vi "Track3.vi"() -> ()   [LabVIEW 2011]
doc: "This VI demonstrates how to control the Robotics Starter Kit 1.0 robot. It is deployed to an sbRIO-9631, then run on the Real-Time controller."
uses:
  <vilib>/Analysis/Matrix/Datatypes/RealMatrix.ctl
  <vilib>/Platform/TimedLoop/XDataNode/timing_clust.ctl
  <vilib>/Platform/TimedLoop/XDataNode/nitl_modes.ctl
  <vilib>/Platform/TimedLoop/XDataNode/wakeup.ctl
  <vilib>/robotics/Starter Kit/1.0/9631 Host Interface/NI_Robotics_Starter Kit Host_9631_1.0.lvclass
  <vilib>/Analysis/Matrix/Numeric/Conversions/Array To Matrix - RA.vi
  <vilib>/Platform/TimedLoop/XDataNode/XDataNode.xnode
  <vilib>/Platform/TimedLoop/XDataNode/XDNodeRunTimeDep.lvlib
  <vilib>/Analysis/Matrix/NI_Matrix.lvlib
  <vilib>/robotics/Starter Kit/Host Interface/NI_Robotics_Starter Kit Host.lvclass
panel:
  out "X-Y 4":cluster{dbl[], dbl[]}(graph)
  out "W":cluster{dbl[], dbl[]}(graph)
  out "VL":cluster{dbl[], dbl[]}(graph)
  in  "Kp W":dbl step=0.01
  in  "Kp VL":dbl step=0.01
  in  "Paso":dbl
  in  "Tiempo":dbl
  in  "stop":bool
  out "X-Y":cluster{dbl[], dbl[]}(graph)
  out "Error":T1
  out "Xr - X":dbl[](array[numeric])
  out "Zigma":dbl[](array[numeric])
  out "Zigmar":dbl[](array[numeric])
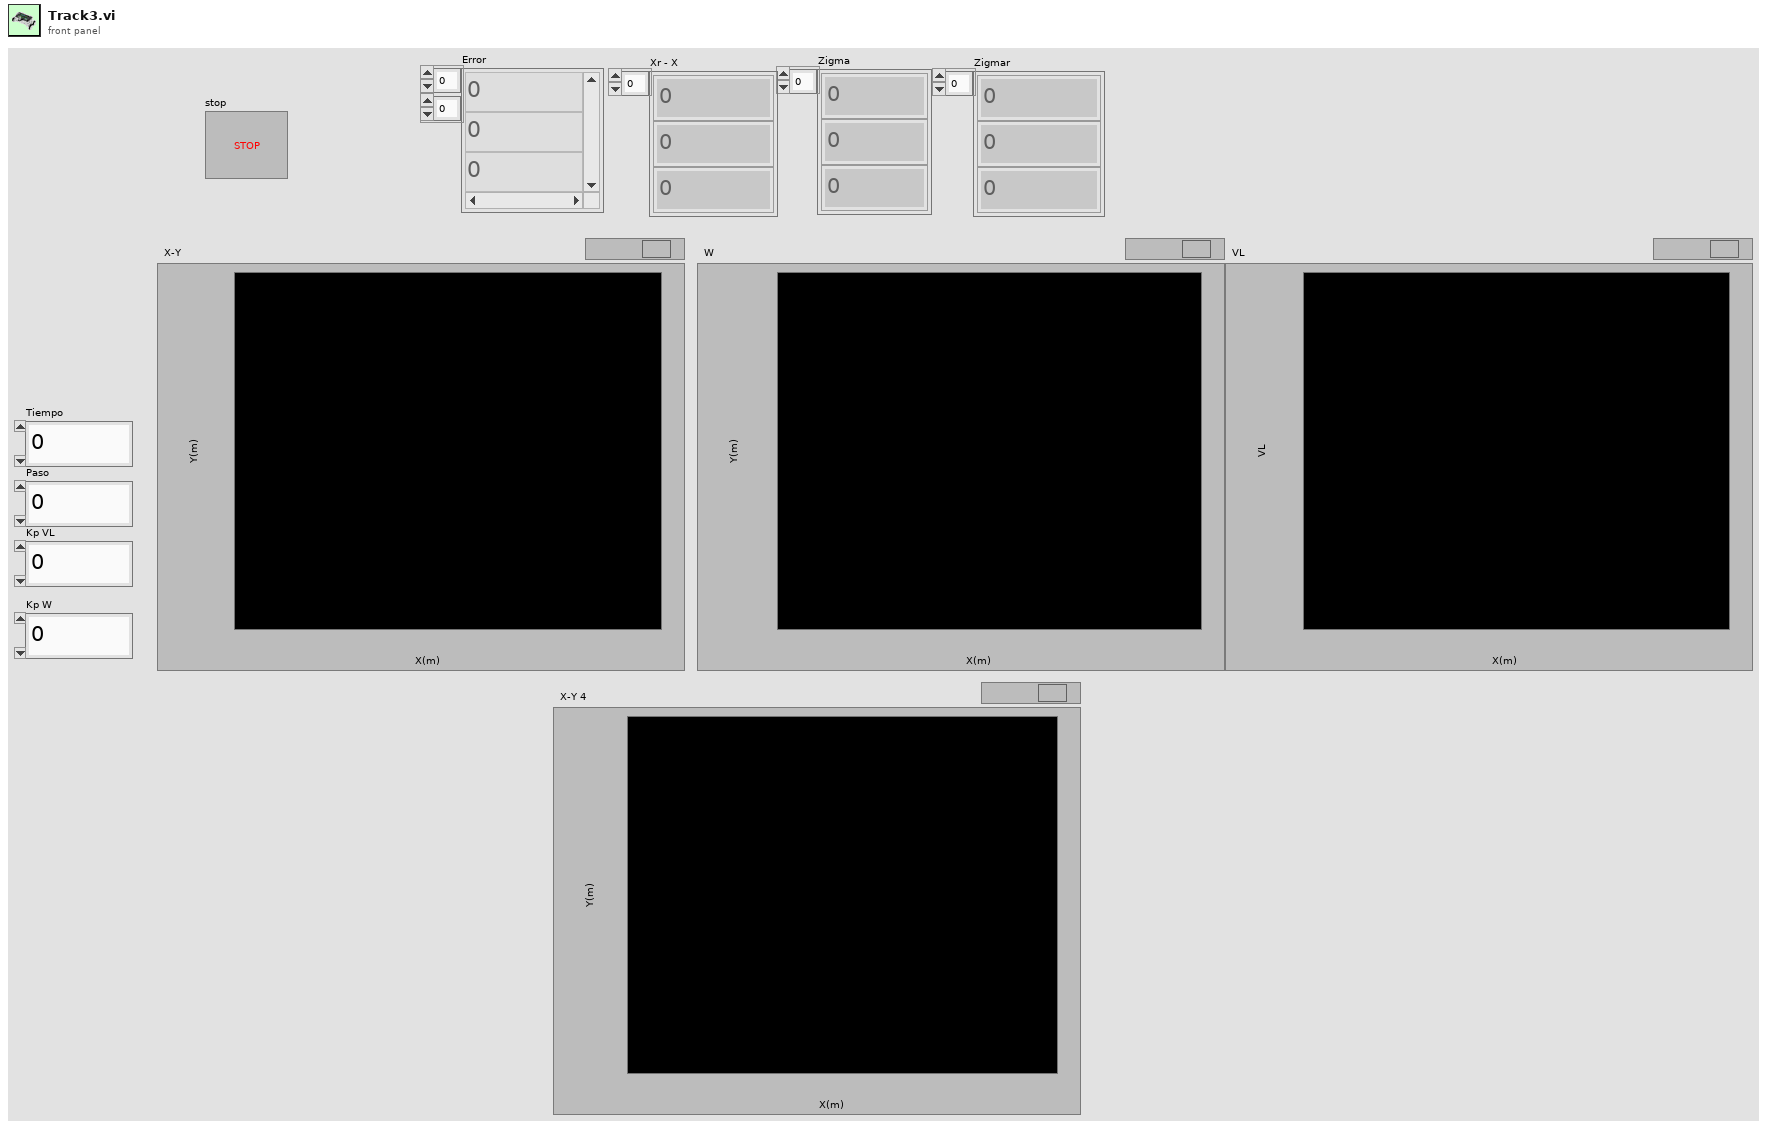
[diagram p1: front panel]
types:
  T1 = typedef "NI_Matrix.lvlib/RealMatrix.ctl" = dbl[][]
  T2 = typedef "XDNodeRunTimeDep.lvlib/timing_clust.ctl" = cluster{"Expected End [f-1]":u64, "Actual End [f-1]":u64, "Finished Late? [f-1]":bool, "Expected End [i-1]":u64, "Actual End [i-1]":u64, "Finished Late? [i-1]":bool, "Expected Start [i]":u64, "Actual Start [i]":u64, "Expected Start [f]":u64, "Actual Start [f]":u64, "Source Name":string, "Structure Name":string, "Period":i64, "Deadline":i64, "Offset":i64, "Start":i64, "Priority":i32, "Timeout":i32, "Mode":T3, "Wakeup Reason":T4, "Error":errorcluster, "Source Type":string, "Secondary Source Type":string, "Global End Time":u64, "Global Start Time":u64, "Frame Duration":u64, "Iteration Duration":u64, "Assigned CPU":i32, "I/O Scan Engine Mode":u32}
  T3 = typedef "XDNodeRunTimeDep.lvlib/nitl_modes.ctl" = enum32{"No Change", "Process missed periods, maintain original phase", "Discard missed periods, maintain original phase", "Process missed periods, ignore original phase", "Discard missed periods, ignore original phase"}
  T4 = typedef "XDNodeRunTimeDep.lvlib/wakeup.ctl" = enum32{"Normal", "Aborted", "Asynchronous wakeup", "Timing source error", "Timed loop error", "Timeout"}
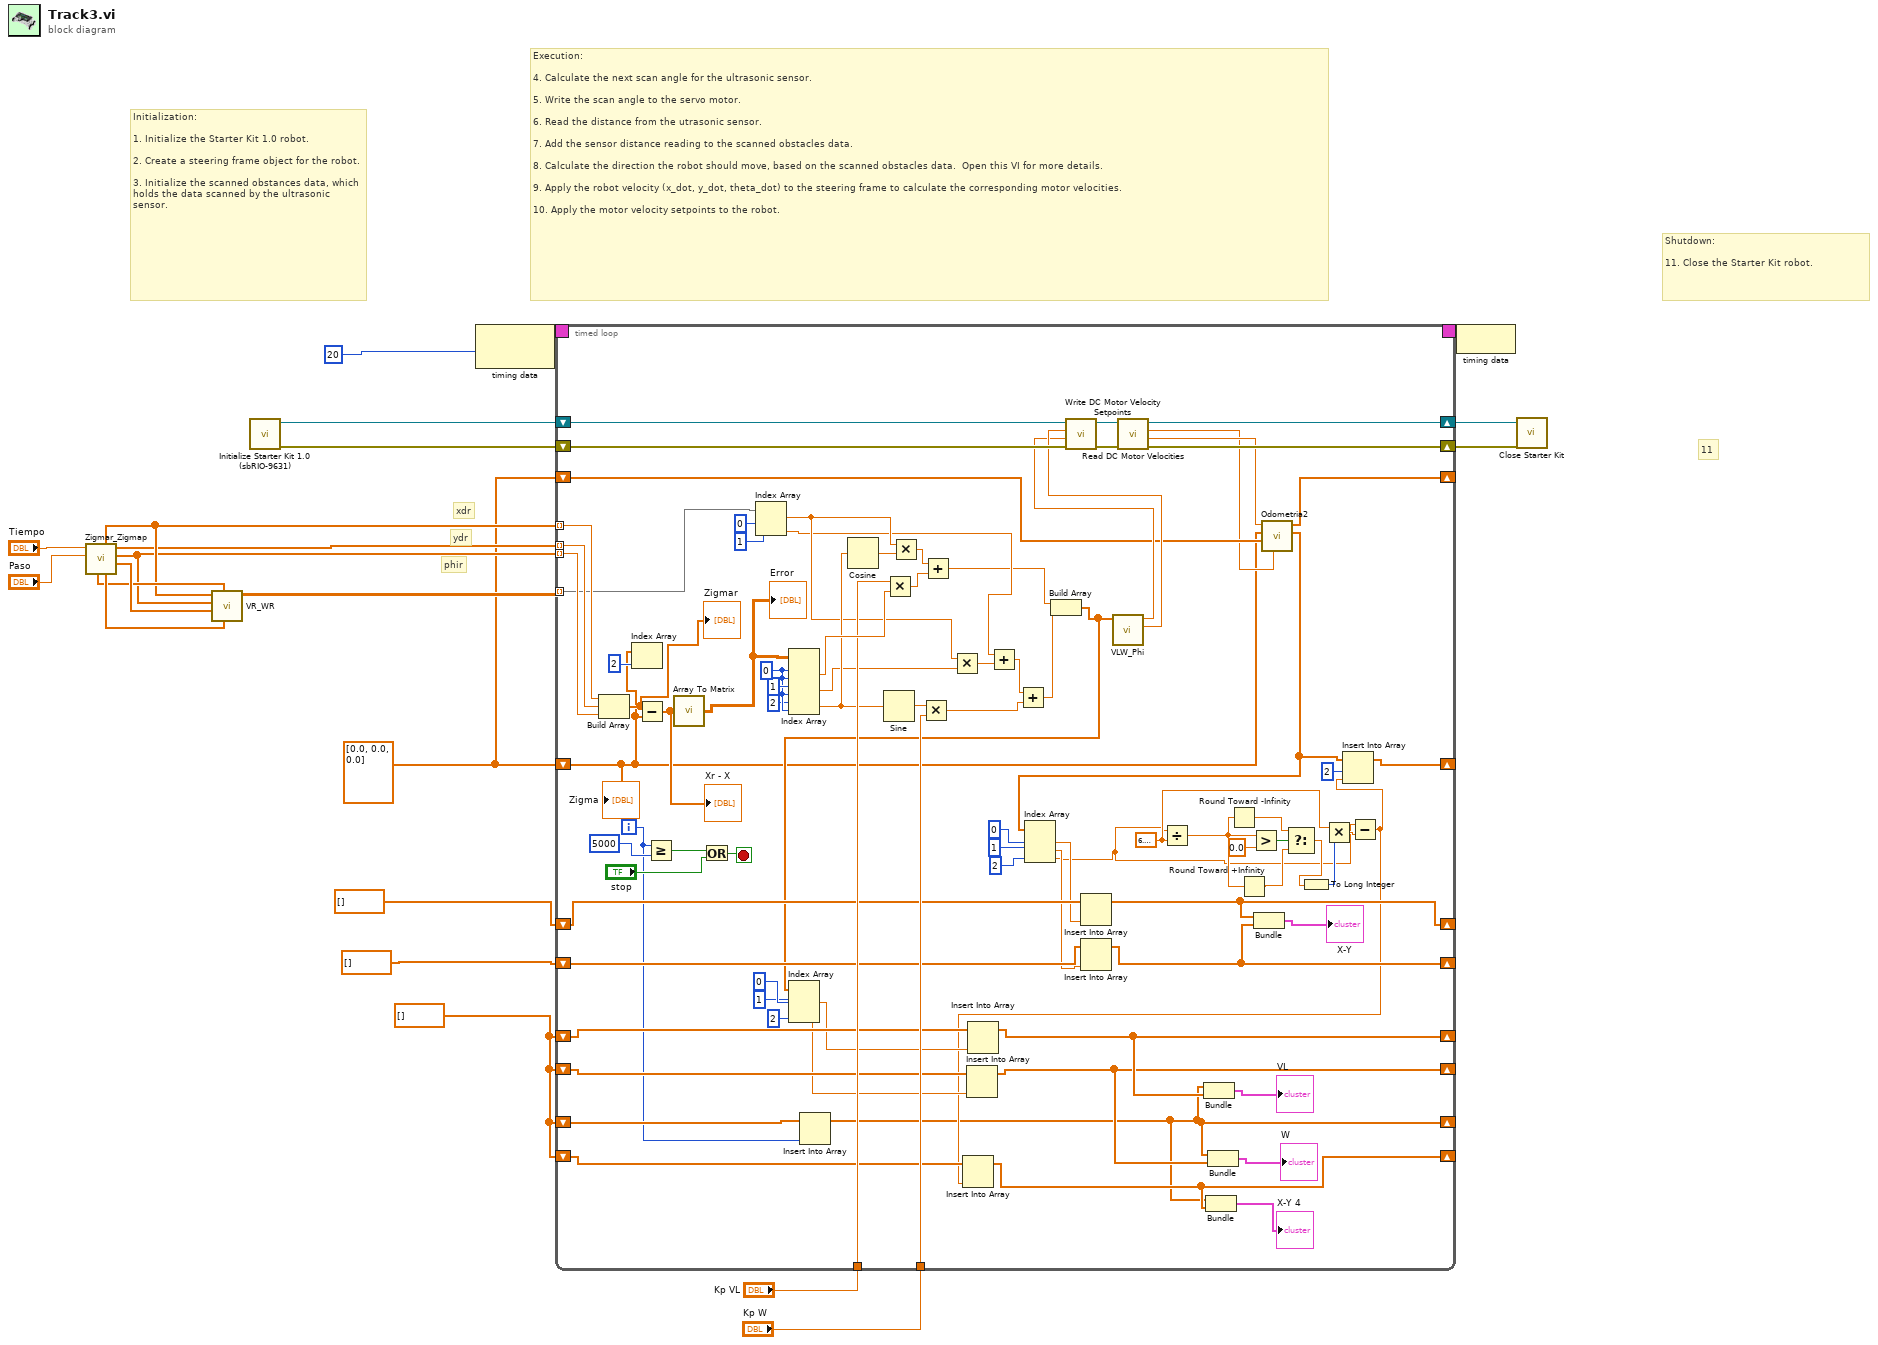
[diagram p0: block diagram]
diagram:
  w1 = dbl[] []
  w8 = dbl[] [0.0, 0.0, 0.0]
  # "phir"
  # "ydr"
  # "xdr"
  # "11"
  # "Shutdown:\n\n11. Close the Starter Kit robot."
  # "Execution:\n\n4. Calculate the next scan angle for the ultrasonic sensor.\n\n5. Write the scan angle to the servo motor.\n\n6. Read the distance from the utrasonic sensor.\n\n7. Add the sensor distance reading to the scanned obstacles data.\n\n8. Calculate the direction the robot should move, based on the scanned obstacles data.  Open this VI for more details.\n\n9. Apply the robot velocity (x_dot, y_dot, theta_dot) to the steering frame to calculate the corresponding motor velocities.\n\n10. Apply the motor velocity setpoints to the robot."
  # "Initialization:\n\n1. Initialize the Starter Kit 1.0 robot.\n\n2. Create a steering frame object for the robot.\n\n3. Initialize the scanned obstances data, which holds the data scanned by the ultrasonic sensor."
  n1 = call "Zigmar_Zigmap.vi"("Paso"="Paso", "Tiempo"="Tiempo") -> ("Xdrp"=w16:dbl[], "Phir"=w11:dbl[], "Ydr"=w12:dbl[], "Ydrp"=w17:dbl[], "Xdr"=w13:dbl[], "Phirp"=w15:dbl[])  [unwired: 4 in]
  n2 = call "VR_WR.vi"("Ydrp"=w17, "Phirp"=w15, "Xdrp"=w16, "Phir"=w11, "Xdr"=w13) -> ("Array"=w14:dbl[][])  [unwired: 6 in]
  n3 = call <vilib>:"Initialize Starter Kit 1.0 (sbRIO-9631).vi"() -> ("error out"=w5:errorcluster, "FPGA starter kit host 1.0 out"=w4:refnum<class "NI_Robotics_Starter Kit Host_9631_1.0.lvclass">)  [unwired: 10 in]
  n4 = node-c288(i64 20 ("Period")) -> (w22:T2)
  n5 = timed-loop {
    shift-right: [w77] -> w2
    shift-left: w4 -> [w79]
    shift-right: [w76] -> w3
    shift-left: w5 -> [w78]
    timing: w22 -> [_]
    timing-out: [_] -> w21
    tunnel: w14 -> [w101] mode=indexing
    tunnel: w13 -> [w110] mode=indexing
    tunnel: w12 -> [w109] mode=indexing
    tunnel: w11 -> [w108] mode=indexing
    shift-right: [w56] -> _
    shift-left: w8 -> [w24]
    tunnel: "Kp VL" -> [w96]
    tunnel: "Kp W" -> [w90]
    shift-right: [w70] -> _
    shift-left: w8 -> [w71]
    shift-right: [w63] -> _
    shift-left: dbl[] [] -> [w69]
    shift-right: [w62] -> _
    shift-left: dbl[] [] -> [w65]
    shift-right: [w35] -> _
    shift-left: w1 -> [w44]
    shift-right: [w30] -> _
    shift-left: w1 -> [w39]
    shift-right: [w26] -> _
    shift-left: w1 -> [w34]
    shift-right: [w29] -> _
    shift-left: w1 -> [w32]
    i -> [w33]
    stop <- w106 stop-if-true
    w55 = 6.283185307179586
    w99 = 0 ("index (row)")
    n6 = Build Array(w110, w109, w108) -> (w28:dbl[])
    "Zigmar" <- w28
    n7 = Index Array(array=w24, index=2) -> ()  [unwired: 1 out]
    n8 = Subtract(x=w28, y=w24) -> (x-y=w104:dbl[])
    "Xr - X" <- w104
    n9 = Greater Or Equal?(x=w33, y=5000 ("x")) -> (x >= y?=w72:bool)
    n10 = call-poly <vilib>:"Array To Matrix.vi"("Real 1D Array"=w104) -> ("Real Matrix (Column Vector)"=w23:T1)
    "Error" <- w23
    n11 = Or(x=w72, y="stop") -> (x .or. y?=w106:bool)
    n12 = Index Array(array=w101, index #1=0 ("index"), index #2=1 ("index")) -> (element #1=w85:dbl, element #2=w84:dbl)
    n13 = Index Array(array=w23, index (row) #1=w99, index (col) #1=w99, index (row) #2=1 ("index (row)"), index (col) #2=w99, index (row) #3=2 ("index (row)"), index (col) #3=w99) -> (element #1=w97:dbl, element #2=w86:dbl, element #3=w92:dbl)
    n14 = Insert Into Array(array=w34, new element=w33) -> (w26:dbl[])  [unwired: 1 in]
    n15 = Cosine(x=w92) -> (cos(x)=w95:dbl)
    n16 = Sine(x=w92) -> (sin(x)=w91:dbl)
    n17 = Multiply(x=w96, y=w97) -> (x*y=w94:dbl)
    n18 = Multiply(x=w85, y=w95) -> (x*y=w93:dbl)
    n19 = Multiply(x=w91, y=w90) -> (x*y=w87:dbl)
    n20 = Add(x=w93, y=w94) -> (x+y=w83:dbl)
    n21 = Multiply(x=w85, y=w86) -> (x*y=w89:dbl)
    n22 = Add(x=w84, y=w89) -> (x+y=w88:dbl)
    n23 = Add(x=w88, y=w87) -> (x+y=w82:dbl)
    n24 = Build Array(w83, w82) -> (w43:dbl[])
    n25 = Index Array(array=w43, index #1=0 ("index"), index #2=1 ("index"), index #3=2 ("index")) -> (element #1=w40:dbl, element #2=w38:dbl)  [unwired: 1 out]
    n26 = Insert Into Array(array=w39, new element=w38) -> (w30:dbl[])  [unwired: 1 in]
    n27 = Insert Into Array(array=w44, new element=w40) -> (w35:dbl[])  [unwired: 1 in]
    n28 = call "VLW_Phi.vi"("VL/W"=w43) -> ("PhiL"=w75:dbl, "PhiR"=w74:dbl)  [unwired: 9 in]
    n29 = call <vilib>:"Write DC Motor Velocity Setpoints.vi"("error in (no error)"=w78, "right motor ccw velocity (rad/s)"=w74, "left motor ccw velocity (rad/s)"=w75, "starter kit host in"=w79) -> ("error out"=w81:errorcluster, "starter kit host out"=w80:refnum<class "NI_Robotics_Starter Kit Host_9631_1.0.lvclass">)  [unwired: 6 in]
    n30 = call <vilib>:"Read DC Motor Velocities.vi"("error in (no error)"=w81, "starter kit host in"=w80) -> ("error out"=w76:errorcluster, "right motor ccw velocity (rad/s)"=w60:dbl, "left motor ccw velocity (rad/s)"=w59:dbl, "starter kit host out"=w77:refnum<class "NI_Robotics_Starter Kit Host_9631_1.0.lvclass">)  [unwired: 6 in]
    n31 = Bundle(w26, w35) -> (→"VL":cluster{dbl[], dbl[]})  [unwired: 1 in]
    n32 = Bundle(w26, w30) -> (→"W":cluster{dbl[], dbl[]})  [unwired: 1 in]
    n33 = call "Odometria2.vi"("left motor ccw velocity (rad/s)"=w59, "Arrastrado"=w71, "Zigma"=w24, "right motor ccw velocity (rad/s)"=w60) -> ("Array out"=w57:dbl[], "Arrastrad_out"=w70:dbl[])  [unwired: 6 in]
    n34 = Index Array(array=w57, index #1=0 ("index"), index #2=1 ("index"), index #3=2 ("index")) -> (element #1=w66:dbl, element #2=w64:dbl, element #3=w46:dbl)
    n35 = Insert Into Array(array=w69, new element=w66) -> (w63:dbl[])  [unwired: 1 in]
    n36 = Insert Into Array(array=w65, new element=w64) -> (w62:dbl[])  [unwired: 1 in]
    n37 = Divide(x=w46, y=w55) -> (x/y=w50:dbl)
    n38 = Round Toward -Infinity(1:w50) -> (0:w52:dbl)
    n39 = Round Toward +Infinity(x=w50) -> (ceil(x): smallest int >= x=w49:dbl)
    n40 = Greater?(x=w50, y=0.0) -> (0:w54:bool)
    n41 = Bundle(w63, w62) -> (→"X-Y":cluster{dbl[], dbl[]})  [unwired: 1 in]
    n42 = Select(t=w52, s=w54, f=w49) -> (s? t:f=w47:dbl)
    n43 = To Long Integer(number=w47) -> (32bit integer=w48:i32)
    n44 = Multiply(x=w55, y=w48) -> (x*y=w53:dbl)
    n45 = Subtract(x=w46, y=w53) -> (x-y=w27:dbl)
    n46 = Insert Into Array(array=w32, new element=w27) -> (w29:dbl[])  [unwired: 1 in]
    n47 = Bundle(w26, w29) -> (→"X-Y 4":cluster{dbl[], dbl[]})  [unwired: 1 in]
    n48 = Insert Into Array(array=w57, index=2, new element=w27) -> (w56:dbl[])
    "Zigma" <- w24
  }
  n49 = node-c288(w21) -> ()
  n50 = call-dynamic "Close Starter Kit.vi"("error in (no error)"=w3, "starter kit host in"=w2) -> ()  [unwired: 9 in, 1 out]
